vi "CVT2GroupWriteTest.vi"() -> (3 "Unit Test Framework Results":T1)   [LabVIEW 2013, in "UnitTests.lvlib"]
uses:
  UnitTests.lvlib
  <vilib>/utf/common/utf_test_result_troll.ctl
  <vilib>/utf/common/utf_test_result.ctl
  <vilib>/utf/common/utf_test_result_failure.ctl
  <vilib>/utf/common/utf_test_comparison_operators.ctl
  <vilib>/utf/common/utf_vi_tag.ctl
  <vilib>/NI/Current Value Table/Type Defs/Group Data.ctl
  <vilib>/NI/Current Value Table/Write grouped data to tags.vi
  <vilib>/NI/Current Value Table/Read tags into grouped data.vi
  <vilib>/NI/Current Value Table/Write Index Set.vi
  <vilib>/NI/Current Value Table/DataTypes/Double_Write Index Set.vi
  <vilib>/NI/Current Value Table/DataTypes/Array of String_Write Index Set.vi
  <vilib>/NI/Current Value Table/DataTypes/Array of Boolean_Write Index Set.vi
  <vilib>/NI/Current Value Table/DataTypes/Array of Single_Write Index Set.vi
  <vilib>/NI/Current Value Table/DataTypes/Array of Double_Write Index Set.vi
  <vilib>/NI/Current Value Table/DataTypes/Array of I8_Write Index Set.vi
  <vilib>/NI/Current Value Table/DataTypes/Array of I16_Write Index Set.vi
  <vilib>/NI/Current Value Table/DataTypes/Array of I32_Write Index Set.vi
  <vilib>/NI/Current Value Table/DataTypes/Array of I64_Write Index Set.vi
  <vilib>/NI/Current Value Table/DataTypes/Array of U64_Write Index Set.vi
  <vilib>/NI/Current Value Table/DataTypes/Array of U32_Write Index Set.vi
  <vilib>/NI/Current Value Table/DataTypes/Array of U16_Write Index Set.vi
  <vilib>/NI/Current Value Table/DataTypes/Array of U8_Write Index Set.vi
  <vilib>/NI/Current Value Table/DataTypes/Boolean_Write Index Set.vi
  <vilib>/NI/Current Value Table/DataTypes/String_Write Index Set.vi
  <vilib>/NI/Current Value Table/DataTypes/U8_Write Index Set.vi
  <vilib>/NI/Current Value Table/DataTypes/U16_Write Index Set.vi
  <vilib>/NI/Current Value Table/DataTypes/U32_Write Index Set.vi
  <vilib>/NI/Current Value Table/DataTypes/U64_Write Index Set.vi
  <vilib>/NI/Current Value Table/DataTypes/I8_Write Index Set.vi
  <vilib>/NI/Current Value Table/DataTypes/I16_Write Index Set.vi
  <vilib>/NI/Current Value Table/DataTypes/I32_Write Index Set.vi
  <vilib>/NI/Current Value Table/DataTypes/I64_Write Index Set.vi
  <vilib>/NI/Current Value Table/DataTypes/Single_Write Index Set.vi
  <vilib>/NI/Current Value Table/Read Index Set.vi
  <vilib>/NI/Current Value Table/DataTypes/Double_Read Index Set.vi
  <vilib>/NI/Current Value Table/DataTypes/Array of String_Read Index Set.vi
  <vilib>/NI/Current Value Table/DataTypes/Array of Boolean_Read Index Set.vi
  <vilib>/NI/Current Value Table/DataTypes/Array of Single_Read Index Set.vi
  <vilib>/NI/Current Value Table/DataTypes/Array of Double_Read Index Set.vi
  <vilib>/NI/Current Value Table/DataTypes/Array of I8_Read Index Set.vi
  <vilib>/NI/Current Value Table/DataTypes/Array of I16_Read Index Set.vi
  <vilib>/NI/Current Value Table/DataTypes/Array of I32_Read Index Set.vi
  <vilib>/NI/Current Value Table/DataTypes/Array of I64_Read Index Set.vi
  <vilib>/NI/Current Value Table/DataTypes/Array of U64_Read Index Set.vi
  <vilib>/NI/Current Value Table/DataTypes/Array of U32_Read Index Set.vi
  <vilib>/NI/Current Value Table/DataTypes/Array of U16_Read Index Set.vi
  <vilib>/NI/Current Value Table/DataTypes/Array of U8_Read Index Set.vi
  <vilib>/NI/Current Value Table/DataTypes/Boolean_Read Index Set.vi
  <vilib>/NI/Current Value Table/DataTypes/String_Read Index Set.vi
  <vilib>/NI/Current Value Table/DataTypes/U8_Read Index Set.vi
  <vilib>/NI/Current Value Table/DataTypes/U16_Read Index Set.vi
  <vilib>/NI/Current Value Table/DataTypes/U32_Read Index Set.vi
  <vilib>/NI/Current Value Table/DataTypes/U64_Read Index Set.vi
  <vilib>/NI/Current Value Table/DataTypes/I8_Read Index Set.vi
  <vilib>/NI/Current Value Table/DataTypes/I16_Read Index Set.vi
  <vilib>/NI/Current Value Table/DataTypes/I32_Read Index Set.vi
  <vilib>/NI/Current Value Table/DataTypes/I64_Read Index Set.vi
  <vilib>/NI/Current Value Table/DataTypes/Single_Read Index Set.vi
  <vilib>/NI/Current Value Table/FGVs/Group Memory.vi
  <vilib>/NI/Current Value Table/Memory Block.vi
  <vilib>/NI/Current Value Table/DataTypes/Double_Memory Block.vi
  <vilib>/NI/Current Value Table/DataTypes/Array of String_Memory Block.vi
  <vilib>/NI/Current Value Table/DataTypes/Array of Boolean_Memory Block.vi
  <vilib>/NI/Current Value Table/DataTypes/Array of Single_Memory Block.vi
  <vilib>/NI/Current Value Table/DataTypes/Array of Double_Memory Block.vi
  <vilib>/NI/Current Value Table/DataTypes/Array of I8_Memory Block.vi
  <vilib>/NI/Current Value Table/DataTypes/Array of I16_Memory Block.vi
  <vilib>/NI/Current Value Table/DataTypes/Array of I32_Memory Block.vi
  <vilib>/NI/Current Value Table/DataTypes/Array of I64_Memory Block.vi
  <vilib>/NI/Current Value Table/DataTypes/Array of U64_Memory Block.vi
  <vilib>/NI/Current Value Table/DataTypes/Array of U32_Memory Block.vi
  <vilib>/NI/Current Value Table/DataTypes/Array of U16_Memory Block.vi
  <vilib>/NI/Current Value Table/DataTypes/Array of U8_Memory Block.vi
  <vilib>/NI/Current Value Table/DataTypes/Boolean_Memory Block.vi
  <vilib>/NI/Current Value Table/DataTypes/String_Memory Block.vi
  <vilib>/NI/Current Value Table/DataTypes/U8_Memory Block.vi
  <vilib>/NI/Current Value Table/DataTypes/U16_Memory Block.vi
  <vilib>/NI/Current Value Table/DataTypes/U32_Memory Block.vi
  <vilib>/NI/Current Value Table/DataTypes/U64_Memory Block.vi
  <vilib>/NI/Current Value Table/DataTypes/I8_Memory Block.vi
  <vilib>/NI/Current Value Table/DataTypes/I16_Memory Block.vi
  <vilib>/NI/Current Value Table/DataTypes/I32_Memory Block.vi
  <vilib>/NI/Current Value Table/DataTypes/I64_Memory Block.vi
  <vilib>/NI/Current Value Table/DataTypes/Single_Memory Block.vi
  <vilib>/utf/NI_UnitTestFramework.lvlib
  <vilib>/NI/Current Value Table/Current Value Table.lvlib
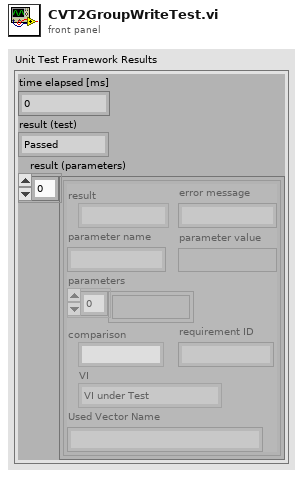
[diagram p1: front panel]
types:
  T1 = typedef "NI_UnitTestFramework.lvlib/utf_test_result_troll.ctl" = cluster{"time elapsed [ms]":u32, "result (test)":T2, "result (parameters)":T3[]}
  T2 = typedef "NI_UnitTestFramework.lvlib/utf_test_result.ctl" = enum16{"Passed", "Failed", "Error", "Skipped", "Not Processed"}
  T3 = typedef "NI_UnitTestFramework.lvlib/utf_test_result_failure.ctl" = cluster{"result":T2, "error message":string, "parameter name":string, "parameter value":variant, "parameters":variant[], "comparison":T4, "requirement ID":string, "VI":T5, "Used Vector Name":string}
  T4 = typedef "NI_UnitTestFramework.lvlib/utf_test_comparison_operators.ctl" = enum16{"=", "!=", ">", ">=", "<", "<=", "range", "symmetric tolerance", "asymmetric tolerance", "string contains", "string not contain", "array size", "string length", "array range", "by element", "array range (limit array)", "user-defined", "array contains", "array not contain", "vector length", "= (elm)", "!= (elm)", "= (case insensitive)", "!= (case insensitive)"}
  T5 = typedef "NI_UnitTestFramework.lvlib/utf_vi_tag.ctl" = enum16{"Setup VI", "VI under Test", "Teardown VI"}
  T6 = typedef "Current Value Table.lvlib/Group Data.ctl" = cluster{"Double":dbl[], "Single":sgl[], "I64":i64[], "I32":i32[], "I16":i16[], "I8":i8[], "U64":u64[], "U32":u32[], "U16":u16[], "U8":u8[], "String":string[], "Boolean":bool[], "Array of U8":cluster{"U8 Array":u8[]}[], "Array of U16":cluster{"U16 Array":u16[]}[], "Array of U32":cluster{"U32 Array":u32[]}[], "Array of U64":cluster{"U64 Array":u64[]}[], "Array of I64":cluster{"I64 Array":i64[]}[], "Array of I32":cluster{"I32 Array":i32[]}[], "Array of I16":cluster{"I16 Array":i16[]}[], "Array of I8":cluster{"I8 Array":i8[]}[], "Array of Double":cluster{"DBL Array":dbl[]}[], "Array of Single":cluster{"SGL Array":sgl[]}[], "Array of Boolean":cluster{"Boolean Array":bool[]}[], "Array of String":cluster{"String Array":string[]}[]}
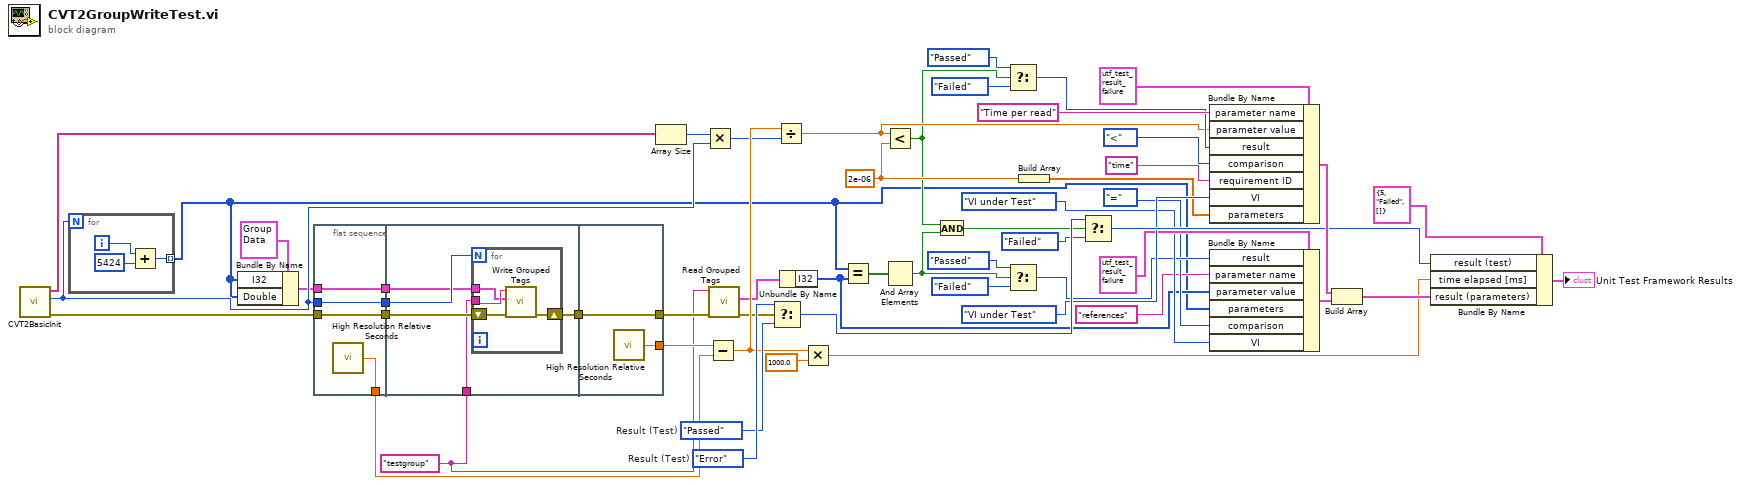
[diagram p0: block diagram]
diagram:
  w2 = "testgroup" ("Group")
  w28 = 2e-06 ("y")
  w49 = utf_test_result."Error"  # Result (Test)
  w48 = utf_test_result."Passed"  # Result (Test)
  n1 = call "CVT2BasicInit.vi"() -> ("error out"=w10:errorcluster, "Tags per type out"=w13:i32, "names"=w23:string[])  [unwired: 9 in]
  n2 = for {
    N: w13 -> [_]
    tunnel: [w55] -> w1 mode=indexing
    i -> [w57]
    n3 = Add(x=w57, y=5424) -> (x+y=w55:i32)
  }
  n4 = Bundle By Name(cluster=T6 {"Double"=[], "Single"=[], "I64"=[], "I32"=[], "I16"=[], "I8"=[], "U64"=[], "U32"=[], "U16"=[], "U8"=[], "String"=[], "Boolean"=[], "Array of U8"=[], "Array of U16"=[], "Array of U32"=[], "Array of U64"=[], "Array of I64"=[], "Array of I32"=[], "Array of I16"=[], "Array of I8"=[], "Array of Double"=[], "Array of Single"=[], "Array of Boolean"=[], "Array of String"=[]} ("Data"), "I32"=w1, "Double"=w1) -> (w7:T6)
  n5 = flat-sequence {
    tunnel: [w61] -> w51
    tunnel: w10 -> [w59]
    tunnel: [w60] -> w43
    tunnel: w13 -> [w60]
    tunnel: [w59] -> w42
    tunnel: [w58] -> w8
    tunnel: w7 -> [w58]
    tunnel: w43 -> [w66]
    tunnel: w42 -> [w65]
    tunnel: [w64] -> w41
    tunnel: w2 -> [w63]
    tunnel: w8 -> [w62]
    tunnel: [w72] -> w52
    tunnel: w41 -> [w71]
    tunnel: [w71] -> w3
    frame #0 {
      n6 = call <vilib>:"High Resolution Relative Seconds.vi"() -> ("relative seconds"=w61:dbl)
    }
    frame #1 {
      n7 = for {
        N: w66 -> [_]
        shift-right: [w69] -> w64
        shift-left: w65 -> [w70]
        tunnel: w63 -> [w68]
        tunnel: w62 -> [w67]
        n8 = call <vilib>:"Write Grouped Tags.vi"("error in (no error)"=w70, "Data"=w67, "Group"=w68) -> ("error out"=w69:errorcluster)  [unwired: 8 in]
      }
    }
    frame #2 {
      n9 = call <vilib>:"High Resolution Relative Seconds.vi"() -> ("relative seconds"=w72:dbl)
    }
  }
  n10 = Array Size(array=w23) -> (size(s)=w22:i32)
  n11 = Multiply(x=w22, y=w13) -> (x*y=w21:i32)
  n12 = Subtract(x=w52, y=w51) -> (x-y=w40:dbl)
  n13 = call <vilib>:"Read Grouped Tags.vi"("error in (no error)"=w3, "Group"=w2) -> ("error out"=w4:errorcluster, "Data"=w6:T6)  [unwired: 8 in]
  n14 = Select(t=w49, s=w4, f=w48) -> (s? t:f=w38:T2)
  n15 = Divide(x=w40, y=w21) -> (x/y=w31:dbl)
  n16 = Unbundle By Name(w6) -> ("I32"=w5:i32[])
  n17 = Multiply(x=w40, y=1000.0) -> (x*y=w44:dbl)
  n18 = Equal?(x=w1, y=w5) -> (x = y?=w12:bool[])
  n19 = Less?(x=w31, y=w28) -> (x < y?=w24:bool)
  n20 = And Array Elements(Boolean array=w12) -> (logical AND=w11:bool)
  n21 = And(x=w24, y=w11) -> (x .and. y?=w25:bool)
  n22 = Select(t=utf_test_result."Passed" ("result"), s=w24, f=utf_test_result."Failed" ("result")) -> (s? t:f=w32:T2)
  n23 = Select(t=utf_test_result."Passed" ("result"), s=w11, f=utf_test_result."Failed" ("result")) -> (s? t:f=w16:T2)
  n24 = Build Array(w28) -> (w27:dbl[])
  n25 = Select(t=w38, s=w25, f=utf_test_result."Failed") -> (s? t:f=w36:T2)
  n26 = Bundle By Name(cluster=T3 {"result"=enum."Passed", "error message"="", "parameter name"="", "parameter value"=variant, "parameters"=[], "comparison"=enum."=", "requirement ID"="", "VI"=enum."Setup VI", "Used Vector Name"=""} ("Unit Test Framework - result (parameters)"), "parameter name"="Time per read", "parameter value"=w31, "result"=w32, "comparison"=utf_test_comparison_operators."<", "requirement ID"="time", "VI"=utf_vi_tag."VI under Test", "parameters"=w27) -> (w47:T3)
  n27 = Bundle By Name(cluster=T3 {"result"=enum."Passed", "error message"="", "parameter name"="", "parameter value"=variant, "parameters"=[], "comparison"=enum."=", "requirement ID"="", "VI"=enum."Setup VI", "Used Vector Name"=""} ("Unit Test Framework - result (parameters)"), "result"=w16, "parameter name"="references" ("format string"), "parameter value"=w5, "parameters"=w1, "comparison"=utf_test_comparison_operators."=", "VI"=utf_vi_tag."VI under Test") -> (w26:T3)
  n28 = Build Array(w47, w26) -> (w46:T3[])
  n29 = Bundle By Name(cluster=T1 {"time elapsed [ms]"=5, "result (test)"=enum."Failed", "result (parameters)"=[]} ("Unit Test Framework - Result"), "result (test)"=w36, "time elapsed [ms]"=w44, "result (parameters)"=w46) -> (→"Unit Test Framework Results":T1)
